vi "Get Assertion Result.vi"(8 "error in (no error)":errorcluster, 11 "Test VIs":T4) -> (0 "error out":errorcluster, 2 "Results":T1[](array[typedef]), 3 "First Result":T1={"Name"="", "Message"="", "Description"="", "Status"=enum."Passed", "Result Type"=enum."Test Suite", "Execution Time"=0.0})   [LabVIEW 2020, in "Compare Assertion Test.lvclass"]
uses:
  Compare Assertion Test.lvclass
  Comparison Test Double/Test Methods.ctl
  source/Core/Result/Result.ctl
  source/Core/Result/Status.ctl
  source/Core/Result/Type.ctl
  Comparison Test Double/Comparison Test Double.lvclass
  C:/git/astemes-lunit/source/API/LUnit Test Case/LUnit Test Case.lvclass
  source/API/LUnit Test Case/LUnit Test Case.lvclass/LUnit Test Case.ctl
  <vilib>/Utility/LVClass/Get LV Class Name.vi
  Compare Assertion Test.lvclass/Compare Assertion Test.ctl
  source/API/LUnit Test Case/LUnit Test Case.lvclass
  C:/git/astemes-lunit/source/Core/Runnable/Runnable.lvclass
  C:/git/astemes-lunit/tests/Comparison Test Double/Comparison Test Double.lvclass
  source/Core/Result/Result.lvlib
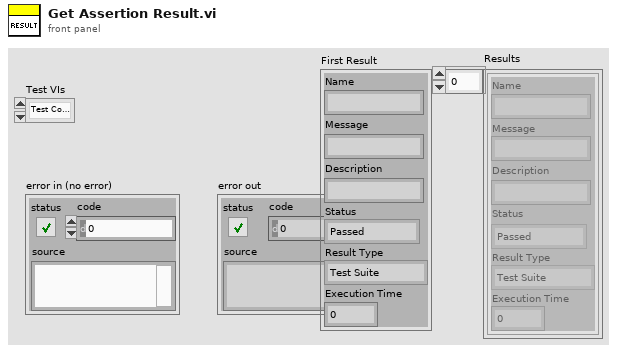
[diagram p1: front panel]
types:
  T1 = typedef "Result.lvlib/Result.ctl" = cluster{"Name":string, "Message":string, "Description":string, "Status":T2, "Result Type":T3, "Execution Time":dbl}
  T2 = typedef "Result.lvlib/Status.ctl" = enum16{"", "Passed", "Failed", "Error", "Skipped", "Setup Error", "Broken", "Teardown Error"}
  T3 = typedef "Result.lvlib/Type.ctl" = enum16{"Test Case", "Test Suite", "Test Run", "Pass", "Fail", "Skip", "Pass if", "Fail if", "Pass if Error", "Fail if Error", "Pass if Equal", "Fail if Equal"}
  T4 = typedef "Comparison Test Double.lvclass/Test Methods.ctl" = enum16{"Test Compare Equal Enums.vi", "Test Compare Unequal Enums.vi", "Test Compare Equal Strings.vi", "Test Compare Unequal Type Deffed Enums.vi", "Test Compare Equal 8bit Enums.vi", "Test Compare Equal 1el String Arrays.vi", "Test Compare Fail if Equal 1el String Arrays.vi"}
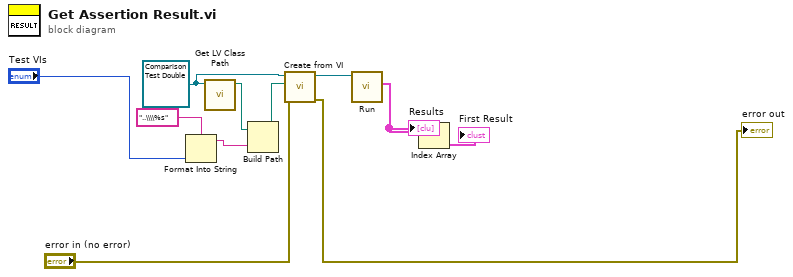
[diagram p0: block diagram]
diagram:
  w2 = refnum<class "Comparison Test Double.lvclass"> refnum ("Comparison Test Double.lvclass")
  n1 = Format Into String(format string="..\\\\%s", "Test VIs") -> (resulting string=w7:string)  [unwired: 2 in, 1 out]
  n2 = call <vilib>:"Get LV Class Path.vi"("object"=w2) -> ("class path"=w4:path)  [unwired: 9 in, 1 out]
  n3 = Build Path(base path=w4, name or relative path=w7) -> (appended path=w1:path)
  n4 = call "Create from VI.vi"("error in (no error)"="error in (no error)", "Test Method VI Path"=w1, "LUnit Test Case Class"=w2) -> ("error out"=→"error out":errorcluster, "LUnit Test Case Out"=w10:refnum<class "Comparison Test Double.lvclass">)  [unwired: 7 in]
  n5 = call-dynamic "Run.vi"("LUnit Test Case In"=w10) -> ("Results"=w11:T1[])  [unwired: 7 in, 3 out]
  "Results" <- w11
  n6 = Index Array(array=w11) -> (element=→"First Result":T1)  [unwired: 1 in]
